vi "Execute Find All Accessors.vi"(6 "Mouse Position":T1, 8 "User VI Ref":refnum<vi>, 9 "Menu Item Tag Suffix":string, 10 "Remaining Items":refnum<vi>[](array[refnum]), 11 "Affected Items":T2) -> (0 "Fail transaction?":bool)   [LabVIEW 2020]
doc: "This VI is part of a plug-in for modifying the LabVIEW shortcut menus. This is the execute VI which is called when the shortcut menu is chosen by the user. It performs the action of the selected menu item."
uses:
  Find All Accessors.ctl
  <vilib>/Utility/miscctls.llb/LVPositionTypeDef.ctl
panel:
  in  "message zero":string="Zero uses of this field found."
  # "All controls on this panel except \"Affected Items\" have been locked to prevent accidental edits. Changing the control names or types, other than the elements of the \"Affected Items\" cluster will make the VI unusable as a menu plugin.\n\nSee Context Help for each control for details about its use."
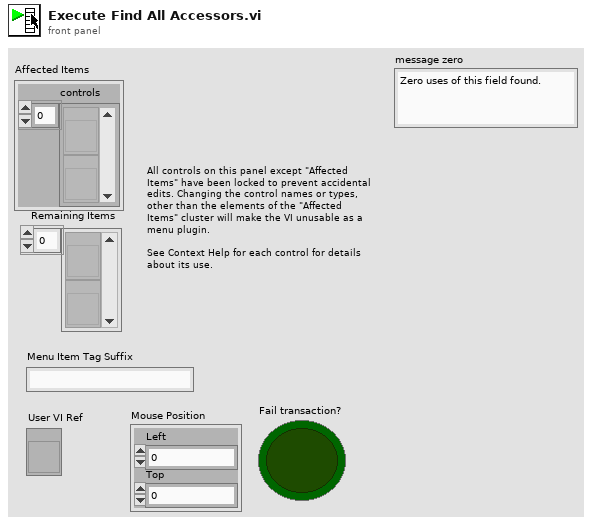
[diagram p1: front panel]
types:
  T1 = typedef "LVPositionTypeDef.ctl" = cluster{"Left":i32, "Top":i32}
  T2 = typedef "Find All Accessors.ctl" = cluster{"controls":refnum<vi>[]}
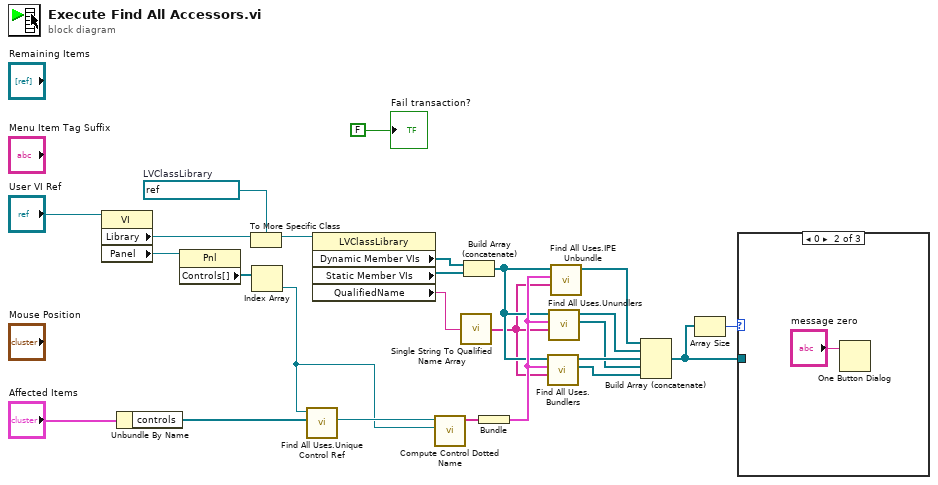
[diagram p0: block diagram]
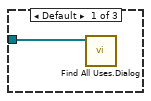
[diagram p2: hidden frame]
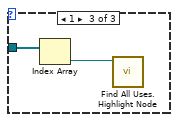
[diagram p3: hidden frame]
diagram:
  w19 = refnum<vi> refnum  # LVClassLibrary
  n1 = property class="VI"(reference="User VI Ref") -> ("Library"=w20:refnum<vi>, "Panel"=w22:refnum<vi>)  [unwired: 1 in, 2 out]
  n2 = Unbundle By Name("Affected Items") -> ("controls"=w5:refnum<vi>[])
  n3 = property class="Pnl"(reference=w22) -> ("Controls[]"=w21:refnum<vi>[])  [unwired: 1 in, 2 out]
  n4 = To More Specific Class(target class=w19, reference=w20) -> (specific class reference=w18:refnum<vi>)  [unwired: 1 in, 1 out]
  n5 = Index Array(array=w21) -> (element=w3:refnum<vi>)  [unwired: 1 in]
  n6 = call "Find All Uses.Unique Control Ref.vi"("controls"=w5, "top cluster"=w3) -> ("selected control"=w4:refnum<vi>)  [unwired: 8 in, 1 out]
  n7 = property class="LVClassLibrary"(reference=w18) -> ("Dynamic Member VIs"=w17:refnum<vi>[], "Static Member VIs"=w16:refnum<vi>[], "QualifiedName"=w14:string)  [unwired: 1 in, 2 out]
  n8 = call "Compute Control Dotted Name.vi"("top control"=w3, "control"=w4) -> ("dotted name"=w15:string[])  [unwired: 9 in]
  n9 = call <vilib>:"Single String To Qualified Name Array.vi"("Fully Qualified String"=w14) -> ("Fully Qualified Array"=w11:string[])
  n10 = Build Array (concatenate)(w17, w16) -> (w12:refnum<vi>[])
  n11 = Bundle("dotted name"=w15) -> (w13:cluster{"dotted name":string[]})  [unwired: 1 in]
  n12 = call "Find All Uses.Bundlers.vi"("Fully Qualified Array"=w11, "dotted name"=w13, "VIs"=w12) -> ("bundle"=w6:refnum<vi>[], "named bundle"=w8:refnum<vi>[])  [unwired: 7 in]
  n13 = call "Find All Uses.Unundlers.vi"("Fully Qualified Array"=w11, "dotted name"=w13, "VIs"=w12) -> ("unbundler"=w7:refnum<vi>[], "named unbundler"=w9:refnum<vi>[])  [unwired: 7 in]
  n14 = call "Find All Uses.IPE Unbundle.vi"("Fully Qualified Array"=w11, "dotted name"=w13, "VIs"=w12) -> ("results"=w10:refnum<vi>[])  [unwired: 8 in]
  n15 = Build Array (concatenate)(w10, w9, w8, w7, w6) -> (w2:refnum<vi>[])
  n16 = Array Size(array=w2) -> (size(s)=w1:i32)
  n17 = case shown="0" w1 {
    tunnel: w2 -> [w26 _ w29]
    frame Default {
      n18 = call "Find All Uses.Dialog.vi"("found"=w26) -> ()  [unwired: 11 in]
    }
    frame 0 {
      n19 = One Button Dialog(message="message zero") -> ()  [unwired: 1 in, 1 out]
    }
    frame 1 {
      n20 = Index Array(array=w29) -> (element=w28:refnum<vi>)  [unwired: 1 in]
      n21 = call "Find All Uses.Highlight Node.vi"("Node in"=w28) -> ()  [unwired: 11 in]
    }
  }
  "Fail transaction?" <- FALSE ("Fail transaction?")
